vi "3.3.vi"() -> ()   [LabVIEW 2017]
panel:
  out "您用时":dbl
  in  "字符串 2":string
  out "开始计时":bool
  in  "长按停止":bool
  # "任务三"
  # "请输入：A virtual instrument is a program in the graphical programming language.\n点击文本框开始计数"
  # "s"
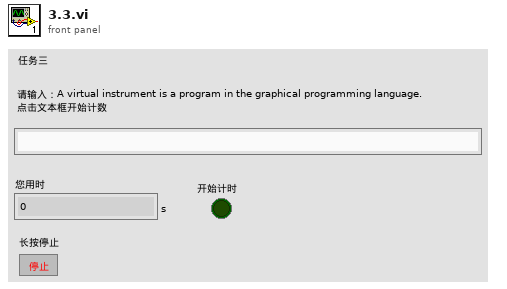
[diagram p1: front panel]
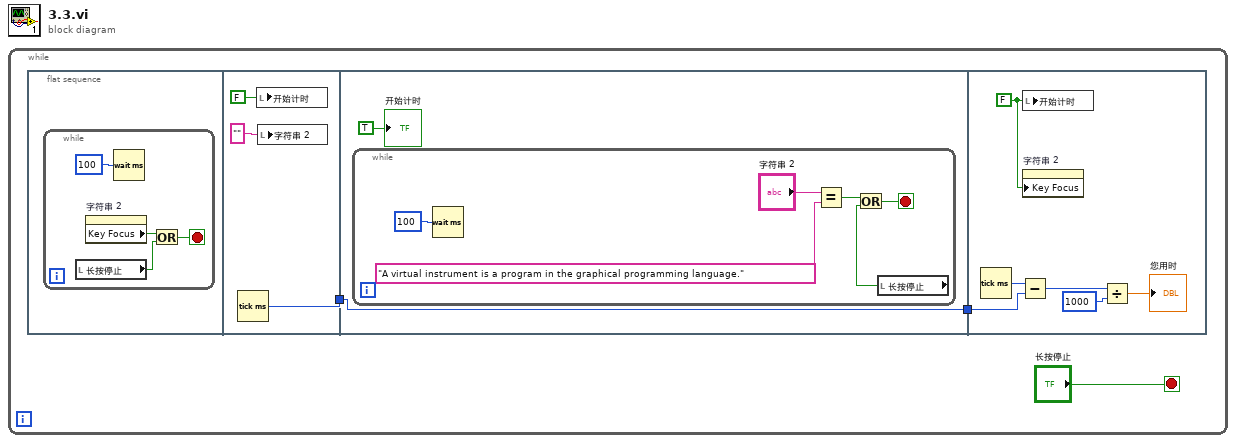
[diagram p0: block diagram]
diagram:
  n1 = while {
    stop <- "长按停止" stop-if-true
    n2 = flat-sequence {
      tunnel: [w9] -> w3
      tunnel: [w12] -> w2
      tunnel: w3 -> [w12]
      tunnel: w2 -> [w23]
      frame #0 {
        n3 = while {
          stop <- w6 stop-if-true
          n4 = local read "长按停止"() -> (w4:bool)
          n5 = property on="字符串 2" class="Str"() -> ("Key Focus"=w5:bool)  [unwired: 2 in, 2 out]
          n6 = Wait (ms)(milliseconds to wait=100) -> ()  [unwired: 1 out]
          n7 = Or(x=w5, y=w4) -> (x .or. y?=w6:bool)
        }
      }
      frame #1 {
        n8 = Tick Count (ms)() -> (millisecond timer value=w9:u32)
        n9 = local write "开始计时"(FALSE) -> ()
        n10 = local write "字符串 2"("") -> ()
      }
      frame #2 {
        n11 = while {
          stop <- w13 stop-if-true
          n12 = Wait (ms)(milliseconds to wait=100) -> ()  [unwired: 1 out]
          n13 = Equal?(x="字符串 2", y="A virtual instrument is a program in the graphical programming language.") -> (x = y?=w15:bool)
          n14 = local read "长按停止"() -> (w14:bool)
          n15 = Or(x=w15, y=w14) -> (x .or. y?=w13:bool)
        }
        "开始计时" <- TRUE
      }
      frame #3 {
        w19 = FALSE
        n16 = Tick Count (ms)() -> (millisecond timer value=w24:u32)
        n17 = Subtract(x=w24, y=w23) -> (x-y=w22:u32)
        n18 = local write "开始计时"(w19) -> ()
        n19 = property on="字符串 2" class="Str"("Key Focus"=w19) -> ()  [unwired: 2 in, 2 out]
        n20 = Divide(x=w22, y=1000) -> (x/y=→"您用时":dbl)
      }
    }
  }
